vi "WordJ.vi"() -> ()   [LabVIEW 2018]
uses:
  <vilib>/Utility/file.llb/Read Delimited Spreadsheet (DBL).vi
panel:
  out "all rows":dbl[][](array[numeric])=[[-3.0, 2.5, -0.75], [-2.99945, 2.50231, -0.75116], [-2.99767, 2.50919, -0.75467], [-2.99427, 2.52049, -0.76053], [-2.98854, 2.53592, -0.76879], [-2.9794, 2.55507, -0.77951], [-2.96526, 2.57733, -0.79277], [-2.9439, 2.60183, -0.80868], [-2.9122, 2.62739, -0.82736], [-2.86594, 2.65231, -0.84901], [-2.79999, 2.67423, -0.87371], [-2.71503, 2.68949, -0.89977], [-2.61151, 2.69666, -0.92672], [-2.48989, 2.69517, -0.95466], [-2.35216, 2.68482, -0.98376], [-2.20174, 2.66574, -1.01419], [-2.04289, 2.63837, -1.04619], [-1.8799, 2.60329, -1.08006], [-1.71643, 2.56105, -1.11624], [-1.55506, 2.51208, -1.15531], [-1.4007, 2.45789, -1.19717], [-1.26457, 2.40356, -1.23909], [-1.14581, 2.35075, -1.28087], [-1.04254, 2.30053, -1.32252], [-0.95305, 2.25375, -1.36406], [-0.87589, 2.21116, -1.40552], [-0.8099, 2.17342, -1.4469], [-0.75417, 2.14113, -1.48823], [-0.70801, 2.11485, -1.52952], [-0.67091, 2.0951, -1.57079], [-0.67091, 2.0951, -1.57079], [-0.66898, 2.08628, -1.57079], [-0.66287, 2.05962, -1.57079], [-0.65172, 2.01452, -1.57079], [-0.6368, 1.95924, -1.57079], [-0.62024, 1.90261, -1.57079], [-0.60211, 1.8445, -1.57079], [-0.5858, 1.79487, -1.57079], [-0.5755, 1.76452, -1.57079], [-0.57198, 1.7543, -1.57079], [-0.57198, 1.7543, -1.57079], [-0.57374, 1.75941, -1.5708], [-0.57897, 1.77468, -1.5708], [-0.58748, 1.79988, -1.5708], [-0.59732, 1.82973, -1.5708], [-0.60678, 1.85917, -1.5708], [-0.61585, 1.88822, -1.5708], [-0.62311, 1.91214, -1.5708], [-0.62733, 1.92637, -1.5708], [-0.62871, 1.9311, -1.5708], [-0.62871, 1.9311, -1.5708], [-0.64821, 1.93827, -1.5708], [-0.70638, 1.95742, -1.5708], [-0.80178, 1.98127, -1.5708], [-0.91228, 1.9963, -1.5708], [-1.01636, 1.9963, -1.5708], [-1.11177, 1.98127, -1.5708], [-1.18324, 1.95742, -1.5708], [-1.22219, 1.93827, -1.5708], [-1.23448, 1.9311, -1.5708], [-1.23448, 1.9311, -1.5708], [-1.23784, 1.93581, -1.5708], [-1.24792, 1.9499, -1.5708], [-1.26476, 1.97318, -1.5708], [-1.28504, 2.00082, -1.5708], [-1.30542, 2.02814, -1.5708], [-1.32592, 2.05515, -1.5708], [-1.34312, 2.07742, -1.5708], [-1.35348, 2.09069, -1.5708], [-1.35695, 2.0951, -1.5708], [-1.35695, 2.0951, -1.5708], [-1.35695, 2.0951, -1.56133], [-1.35695, 2.0951, -1.50808], [-1.35695, 2.0951, -1.39853], [-1.35695, 2.0951, -1.2452], [-1.35695, 2.0951, -1.0756], [-1.35695, 2.0951, -0.92227], [-1.35695, 2.0951, -0.81272], [-1.35695, 2.0951, -0.75947], [-1.35695, 2.0951, -0.75], [-1.35695, 2.0951, -0.75], [-1.35759, 2.09525, -0.75], [-1.3618, 2.09629, -0.75], [-1.37243, 2.09891, -0.75], [-1.39164, 2.10365, -0.75], [-1.42088, 2.11085, -0.75], [-1.46104, 2.12075, -0.75], [-1.51244, 2.13341, -0.75], [-1.5749, 2.14881, -0.75], [-1.64782, 2.16678, -0.75], [-1.73024, 2.18709, -0.75], [-1.82085, 2.20942, -0.75], [-1.91811, 2.23339, -0.75], [-2.02026, 2.25856, -0.75], [-2.1254, 2.28447, -0.75], [-2.23155, 2.31063, -0.75], [-2.33669, 2.33654, -0.75], [-2.43884, 2.36171, -0.75], [-2.5361, 2.38568, -0.75], [-2.62671, 2.40801, -0.75], [-2.70913, 2.42832, -0.75], [-2.78205, 2.44629, -0.75], [-2.84451, 2.46168, -0.75], [-2.89591, 2.47435, -0.75], [-2.93607, 2.48424, -0.75], [-2.96531, 2.49145, -0.75], [-2.98452, 2.49618, -0.75], [-2.99515, 2.49881, -0.75], [-2.99936, 2.49984, -0.75], [-3.0, 2.5, -0.75]]
  in  "file path (dialog if empty)":path=path "/Users/JoshEtkind/Documents/Tufts/Senior Fall/Advanced Robotics/Initials/Physical Robot/wordJ.csv"
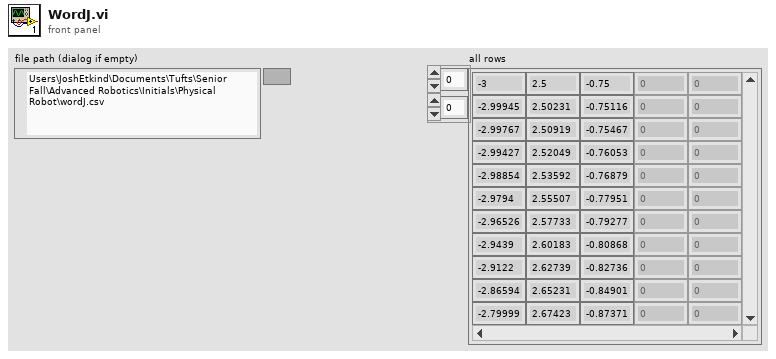
[diagram p1: front panel]
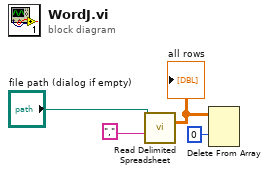
[diagram p0: block diagram]
diagram:
  n1 = call-poly <vilib>:"Read Delimited Spreadsheet.vi"("file path (dialog if empty)"="file path (dialog if empty)", "delimiter (\\t)"="," ("delimiter (\\t)")) -> ("all rows"=w2:dbl[][])  [unwired: 8 in, 5 out]
  "all rows" <- w2
  n2 = Delete From Array(array=w2, index (row)=0) -> ()  [unwired: 2 in, 2 out]
